vi "Ball Stack.vi"(0 "top":bool, 1 "spinOut":bool, 2 "middle":bool, 3 "bottom":bool, 4 "suckMotorSpeed":dbl, 5 "suck":bool, 8 "Vertical Stack Speed":dbl=0.5) -> (6 "topMotor":dbl, 7 "middleMotor":dbl, 9 "bottomMotor":dbl, 10 "suckMotor":dbl)   [LabVIEW 2011]
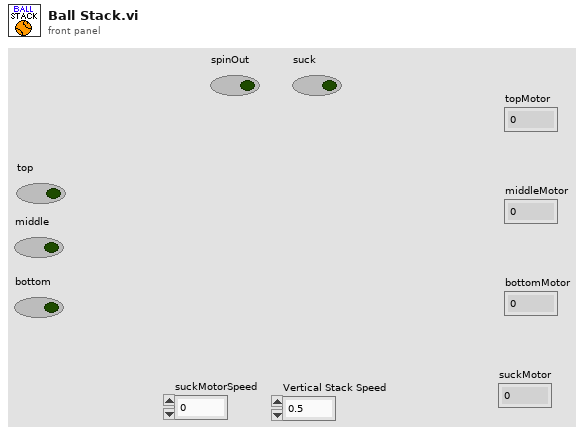
[diagram p1: front panel]
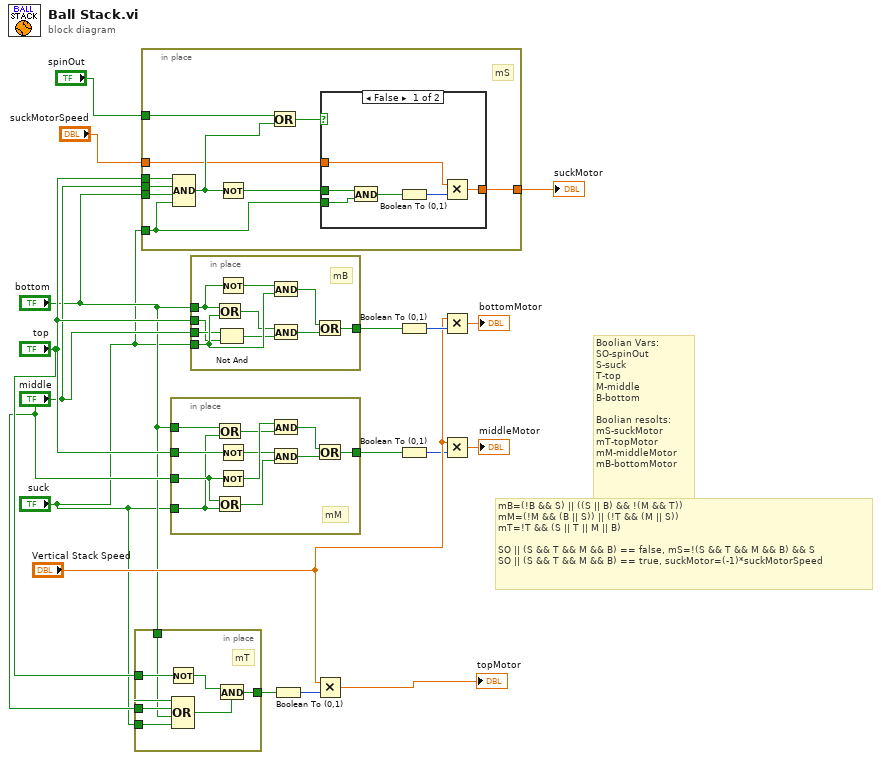
[diagram p0: block diagram]
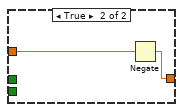
[diagram p2: hidden frame]
diagram:
  # "mB=(!B && S) || ((S || B) && !(M && T))\nmM=(!M && (B || S)) || (!T && (M || S))\nmT=!T && (S || T || M || B)\n\nSO || (S && T && M && B) == false, mS=!(S && T && M && B) && S\nSO || (S && T && M && B) == true, suckMotor=(-1)*suckMotorSpeed"
  # "Boolian Vars:\nSO-spinOut\nS-suck\nT-top\nM-middle\nB-bottom\n\nBoolian resolts:\nmS-suckMotor\nmT-topMotor\nmM-middleMotor\nmB-bottomMotor"
  n1 = in-place {
    in-place-border: [w22] -> w15
    in-place-border: "top" -> [w21]
    in-place-border: "middle" -> [w20]
    in-place-border: "bottom" -> [w19]
    in-place-border: "suck" -> [w18]
    # "mT"
    n2 = Not(x=w21) -> (.not. x?=w24:bool)
    n3 = Compound Arithmetic op=OR(w21, w20, w19, w18) -> (w23:bool)
    n4 = And(x=w24, y=w23) -> (x .and. y?=w22:bool)
  }
  n5 = in-place {
    in-place-border: [w34] -> w17
    in-place-border: "top" -> [w33]
    in-place-border: "middle" -> [w32]
    in-place-border: "bottom" -> [w31]
    in-place-border: "suck" -> [w30]
    in-place-border: "suckMotorSpeed" -> [w26]
    in-place-border: "spinOut" -> [w25]
    # "mS"
    n6 = Compound Arithmetic op=AND(w33, w32, w31, w30) -> (w28:bool)
    n7 = Not(x=w28) -> (.not. x?=w29:bool)
    n8 = Or(x=w25, y=w28) -> (x .or. y?=w27:bool)
    n9 = case shown="False" w27 {
      tunnel: w30 -> [w38 _]
      tunnel: w26 -> [w37 w42]
      tunnel: [w36 w41] -> w34
      tunnel: w29 -> [w35 _]
      frame False {
        n10 = And(x=w35, y=w38) -> (x .and. y?=w40:bool)
        n11 = Boolean To (0,1)(Boolean=w40) -> (0, 1=w39:i16)
        n12 = Multiply(x=w37, y=w39) -> (x*y=w36:dbl)
      }
      frame True {
        n13 = Negate(x=w42) -> (-x=w41:dbl)
      }
    }
  }
  "suckMotor" <- w17
  n14 = in-place {
    in-place-border: "middle" -> [w48]
    in-place-border: "bottom" -> [w51]
    in-place-border: "suck" -> [w47]
    in-place-border: "top" -> [w49]
    in-place-border: [w43] -> w9
    # "mM"
    n15 = Or(x=w51, y=w47) -> (x .or. y?=w52:bool)
    n16 = Or(x=w48, y=w47) -> (x .or. y?=w45:bool)
    n17 = Not(x=w49) -> (.not. x?=w46:bool)
    n18 = Not(x=w48) -> (.not. x?=w53:bool)
    n19 = And(x=w53, y=w52) -> (x .and. y?=w50:bool)
    n20 = And(x=w46, y=w45) -> (x .and. y?=w44:bool)
    n21 = Or(x=w50, y=w44) -> (x .or. y?=w43:bool)
  }
  n22 = in-place {
    in-place-border: "bottom" -> [w61]
    in-place-border: "suck" -> [w60]
    in-place-border: "middle" -> [w57]
    in-place-border: "top" -> [w56]
    in-place-border: [w54] -> w13
    # "mB"
    n23 = Or(x=w61, y=w60) -> (x .or. y?=w58:bool)
    n24 = Not And(1:w56, 2:w57) -> (0:w55:bool)
    n25 = Not(x=w61) -> (.not. x?=w63:bool)
    n26 = And(x=w63, y=w60) -> (x .and. y?=w62:bool)
    n27 = And(x=w58, y=w55) -> (x .and. y?=w59:bool)
    n28 = Or(x=w62, y=w59) -> (x .or. y?=w54:bool)
  }
  n29 = Boolean To (0,1)(Boolean=w15) -> (0, 1=w14:i16)
  n30 = Multiply(x="Vertical Stack Speed", y=w14) -> (x*y=→"topMotor":dbl)
  n31 = Boolean To (0,1)(Boolean=w13) -> (0, 1=w12:i16)
  n32 = Boolean To (0,1)(Boolean=w9) -> (0, 1=w8:i16)
  n33 = Multiply(x="Vertical Stack Speed", y=w12) -> (x*y=→"bottomMotor":dbl)
  n34 = Multiply(x="Vertical Stack Speed", y=w8) -> (x*y=→"middleMotor":dbl)
